vi "Extract Translation.vi"(1 "Transformation matrix":T1) -> (0 "translation":dbl[](array[numeric]))   [LabVIEW 2024]
uses:
  <vilib>/Analysis/Matrix/Datatypes/RealMatrix.ctl
  <vilib>/Analysis/Matrix/NI_Matrix.lvlib
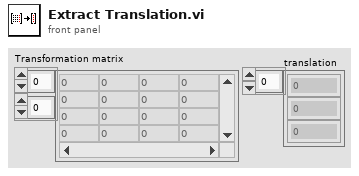
[diagram p1: front panel]
types:
  T1 = typedef "NI_Matrix.lvlib/RealMatrix.ctl" = dbl[][]
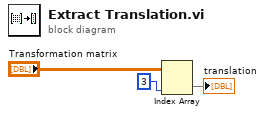
[diagram p0: block diagram]
diagram:
  n1 = Index Array(array="Transformation matrix", index (col)=3 ("disabled index (col)")) -> (element=→"translation":dbl[])  [unwired: 1 in]
